vi "Triax320 VisaRW.vi"(0 "VISA Rsrc":refnum<visa-resource-name>="SR530", 1 "2Lecture?":bool, 2 "EOS (Aucun)":string, 3 "Délais (0 ms)":u32, 5 "ChaineCom":string caption="Chaîne de commande", 9 "Nbcaract":u32=100 caption="Nombre de \ncaractères à lire", 11 "error in (no error)":errorcluster, 12 "Lecture?(T)":bool=TRUE, 13 "Timeout ms":u32=1000) -> (4 "VISA Rsrc Out":refnum<visa-resource-name>="GPIB0::12::INSTR", 6 "ChaineRep":string caption="Chaîne de réponse", 8 "ChaineRep2":string caption="Chaîne de réponse 2", 10 "Count out 2":u32=44 caption="Nombre de caractères lus 2", 14 "Count out":u32=44 caption="Nombre de caractères lus", 15 "error out":errorcluster)   [LabVIEW 2019]
doc: "Ce VI envoie des commande d'écriture et de lecture VISA à l'appareil GPIB. Il permet de ne pas séparer un question de sa réponse. Pour que cela fonctionne toute lecture d'un instrument doit se faire par ce VI."
panel:
  out "Sent Byte 0":u8
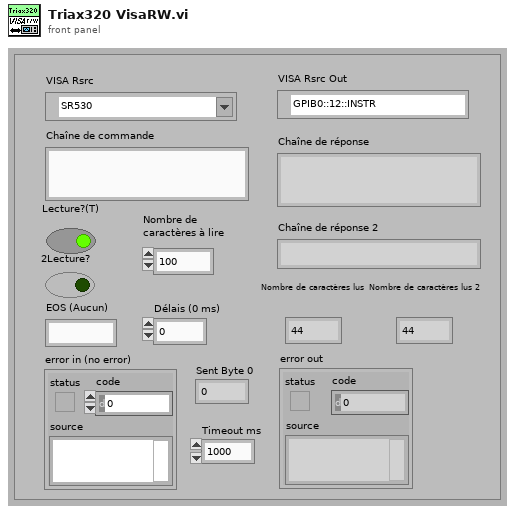
[diagram p1: front panel]
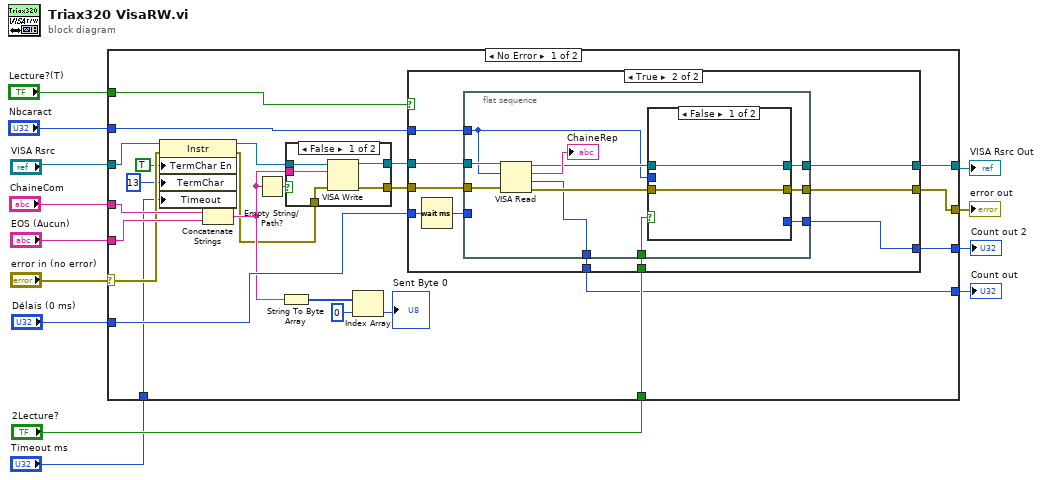
[diagram p0: block diagram]
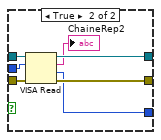
[diagram p4: hidden frame]
diagram:
  n1 = case shown="No Error" "error in (no error)" {
    selector: "error in (no error)" -> [w17 w78]
    tunnel: "VISA Rsrc" -> [w19 w77]
    tunnel: [w37 w77] -> w5
    tunnel: "ChaineCom" -> [w36 _]
    tunnel: "EOS (Aucun)" -> [w35 _]
    tunnel: "Délais (0 ms)" -> [w31 _]
    tunnel: "Nbcaract" -> [w30 _]
    tunnel: "Lecture?(T)" -> [w29 _]
    tunnel: [w34 w78] -> w7
    tunnel: "2Lecture?" -> [w28 _]
    tunnel: [w22 _] -> w3
    tunnel: [w21 _] -> w2
    tunnel: "Timeout ms" -> [w14 _]
    frame No Error {
      n2 = property class="Instr"(reference=w19, error in=w17, "TermChar En"=TRUE ("Message Based Settings:Termination Character Enable"), "TermChar"=u8 13 ("Message Based Settings:Termination Character"), "Timeout"=w14) -> (reference out=w20:refnum<visa-resource-name>, error out=w18:errorcluster)
      n3 = Concatenate Strings(w36, w35) -> (w24:string)
      n4 = Empty String/Path?(string/path=w24) -> (empty?=w23:bool)
      n5 = String To Byte Array(string=w24) -> (unsigned byte array=w27:u8[])
      n6 = case shown="False" w23 {
        tunnel: w20 -> [w42 w44]
        tunnel: w18 -> [w41 w43]
        tunnel: [w40 w44] -> w33
        tunnel: [w39 w43] -> w32
        tunnel: w24 -> [w38 _]
        frame False {
          n7 = VISA Write(VISA resource name=w42, write buffer=w38, error in (no error)=w41) -> (VISA resource name out=w40:refnum<visa-resource-name>, error out=w39:errorcluster)  [unwired: 1 out]
        }
        frame True {
        }
      }
      n8 = Index Array(array=w27, index=0 ("indice")) -> (element=→"Sent Byte 0":u8)
      n9 = case shown="True" w29 {
        tunnel: w33 -> [w46 w56]
        tunnel: [w46 w55] -> w37
        tunnel: w32 -> [w45 w54]
        tunnel: [w45 w53] -> w34
        tunnel: w30 -> [_ w52]
        tunnel: w31 -> [_ w51]
        tunnel: w28 -> [_ w49]
        tunnel: [_ w48] -> w22
        tunnel: [_ w47] -> w21
        frame False {
        }
        frame True {
          n10 = Wait (ms)(milliseconds to wait=w51) -> (millisecond timer value=w50:u32)
          n11 = flat-sequence {
            tunnel: [w63] -> w53
            tunnel: [w61] -> w55
            tunnel: w56 -> [w67]
            tunnel: w54 -> [w65]
            tunnel: w52 -> [w59]
            tunnel: w50 -> [_]
            tunnel: w49 -> [w60]
            tunnel: [w58] -> w48
            tunnel: [w57] -> w47
            frame #0 {
              n12 = VISA Read(VISA resource name=w67, byte count=w59, error in (no error)=w65) -> (VISA resource name out=w62:refnum<visa-resource-name>, read buffer=→"ChaineRep":string, return count=w57:u32, error out=w64:errorcluster)
              n13 = case shown="False" w60 {
                tunnel: w64 -> [w68 w76]
                tunnel: [w68 w75] -> w63
                tunnel: w62 -> [w69 w74]
                tunnel: [w69 w73] -> w61
                tunnel: w59 -> [_ w71]
                tunnel: [_ w70] -> w58
                frame False {
                }
                frame True {
                  n14 = VISA Read(VISA resource name=w74, byte count=w71, error in (no error)=w76) -> (VISA resource name out=w73:refnum<visa-resource-name>, read buffer=→"ChaineRep2":string, return count=w70:u32, error out=w75:errorcluster)
                }
              }
            }
          }
        }
      }
    }
    frame Error {
    }
  }
  "error out" <- w7
  "VISA Rsrc Out" <- w5
  "Count out 2" <- w3
  "Count out" <- w2
